vi "ActorDatabase-UpdateInstructions.vi"(7 "Payload From Actor":string, 8 "error in (no error)":errorcluster, 11 "Database-Actor in":refnum<class "PartCertDatabase-Actor.lvclass">) -> (0 "error out":errorcluster, 2 "JSON Query":string, 3 "Database-Actor out":refnum<class "PartCertDatabase-Actor.lvclass">)   [LabVIEW 2013, in "PartCertDatabase-Actor.lvclass"]
uses:
  PartCertDatabase-Actor.lvclass
  PartCertDatabase-Actor.lvclass/PartCertDatabase-Actor.ctl
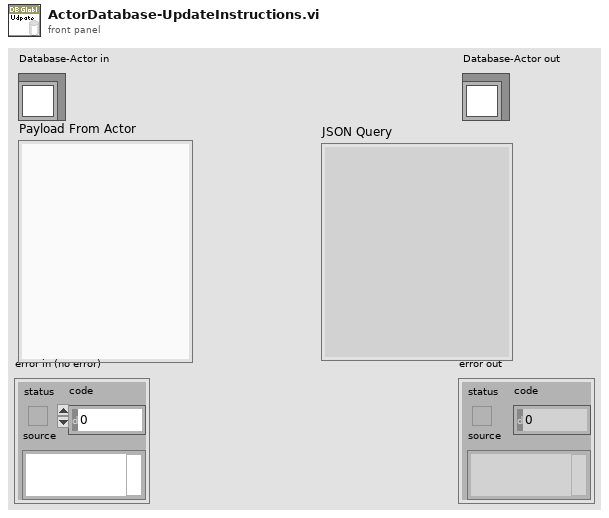
[diagram p1: front panel]
types:
  T1 = cluster{"Table":string, "SQL Statement":string, "Update All":bool, "Payload":string, "Column Number":i32, "Datatype":i32, "Reply Command":string}
  T2 = cluster{"Manufacturing-Part Number":string, "Step Number":string, "Label Instructions":string, "Path for Picture Label":path, "Path for Picture Label 2":path, "Path for Picture Label 3":path, "Path for Picture Label 4":path, "Path for Picture Label 5":path, "Path for Picture Label 6":path, "Path for Picture Label 7":path, "General Instruction Name":string}[]
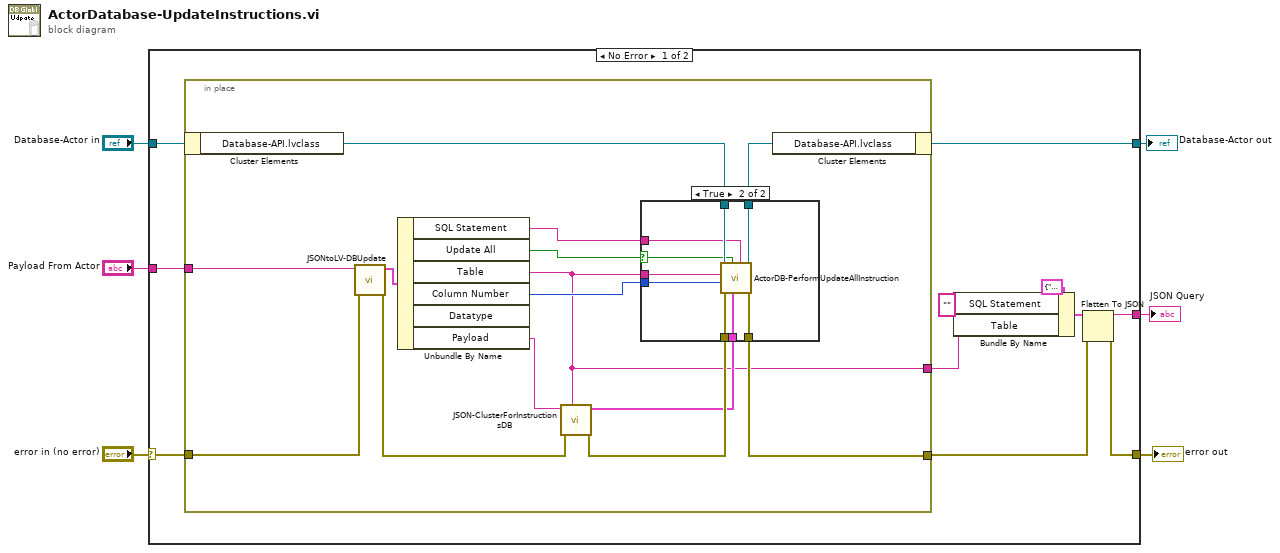
[diagram p0: block diagram]
diagram:
  n1 = case shown="No Error" "error in (no error)" {
    selector: "error in (no error)" -> [w15 w44]
    tunnel: [w9 w44] -> w5
    tunnel: [w16 w43] -> w3
    tunnel: "Database-Actor in" -> [w17 w43]
    tunnel: "Payload From Actor" -> [w14 _]
    tunnel: [w8 _] -> w1
    frame No Error {
      n2 = in-place {
        in-place-border: w15 -> [w28]
        in-place-border: [w20] -> w10
        in-place-border: w14 -> [w19]
        in-place-border: [w18] -> w11
        n3 = in-place-cluster #1(w17) -> ("Database-API.lvclass"=w31:refnum<class "PartCertDatabase-API.lvclass">)
        n4 = call "JSONtoLV-DBUpdate.vi"("error in"=w28, "Input JSON Object"=w19) -> ("error out"=w25:errorcluster, "value"=w27:T1)  [unwired: 8 in]
        n5 = Unbundle By Name(w27) -> ("SQL Statement"=w30:string, "Update All"=w21:bool, "Table"=w18:string, "Column Number"=w29:i32, "Payload"=w26:string)  [unwired: 1 out]
        n6 = call "JSON-ClusterForInstructionsDB.vi"("Table"=w18, "error in (no error)"=w25, "Payload"=w26) -> ("error out"=w24:errorcluster, "Cluster Out"=w23:T2)  [unwired: 7 in]
        n7 = case shown="True" w21 {
          selector: w21 -> [_ w35]
          tunnel: w31 -> [w33 w42]
          tunnel: w30 -> [_ w41]
          tunnel: w18 -> [_ w40]
          tunnel: w29 -> [_ w39]
          tunnel: w24 -> [w32 w38]
          tunnel: w23 -> [_ w37]
          tunnel: [w32 w34] -> w20
          tunnel: [w33 w36] -> w22
          frame False {
          }
          frame True {
            n8 = call "ActorDB-PerformUpdateAllInstruction.vi"("SQL Statement"=w41, "Cluster In"=w37, "Update All"=w35, "error in (no error)"=w38, "Column Number"=w39, "Table"=w40, "Database-API in"=w42) -> ("error out"=w34:errorcluster, "Database-API out"=w36:refnum<class "PartCertDatabase-API.lvclass">)  [unwired: 2 in, 1 out]
          }
        }
        n9 = in-place-cluster #1("Database-API.lvclass"=w22) -> (w16:refnum<class "PartCertDatabase-Actor.lvclass">)
      }
      n10 = Bundle By Name(cluster=cluster{"Table":string, "SQL Statement":string} {"Table"="", "SQL Statement"=""}, "SQL Statement"="", "Table"=w11) -> (w13:cluster{"Table":string, "SQL Statement":string})
      n11 = Flatten To JSON(anything=w13, error in (no error)=w10) -> (JSON string=w8:string, 11:w9:errorcluster)  [unwired: 1 in]
    }
    frame Error {
    }
  }
  "error out" <- w5
  "Database-Actor out" <- w3
  "JSON Query" <- w1
